vi "Humidity Min Read.vi"   [LabVIEW 2023, in "Climate Chamber.lvclass"]
uses:
  Climate Chamber.lvclass
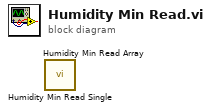
[diagram p0: block diagram]
diagram:
  n1 = call "Humidity Min Read Single.vi"() -> ()  [unwired: 8 in, 4 out]
  n2 = call "Humidity Min Read Array.vi"() -> ()  [unwired: 8 in, 4 out]
